vi "Autonomous Independent.vi"   [LabVIEW 2017]
doc: "This VI is called when autonomous begins, and will automatically be terminated when autonomous ends. You can carry out timed or sensor driven robot movement independently without needing to return to the caller."
uses:
  Autonomous/Enum_AutoAction.ctl
  Autonomous/Enum_AutoState.ctl
  Systems/Gear/ENUM_Servo Position.ctl
  Systems/MechamumDrive/Cluster_CMD to SM Data.ctl
  Systems/MechamumDrive/Enum_SM Cmd Select.ctl
  Systems/Shooter/Cluster_CMD to SM Data.ctl
  Systems/Shooter/ENUM_CMD Select.ctl
  Systems/MechamumDrive/Cluster_SM Status.ctl
  Shared Code/TypeDefs/ENUM_Auto Select.ctl
  <vilib>/Rock Robotics/WPI/DriverStation/WPI_DriverStationAllianceInfo.ctl
  Systems/Sonar/Global_HW_Data Out.vi
  Globals/Global_STOP.vi
  Systems/DashBoardCom/Global_Dashboard Controls.vi
  Systems/MechamumDrive/Global_SM Out Data.vi
  Globals/Global_Alliance.vi
  Systems/Shooter/Global_CMD to SM Data.vi
  Systems/MechamumDrive/Global_CMD to SM Data.vi
  Systems/Gear/Global_CMD to HW.vi
  Systems/Hopper/Global_SM_Data Out.vi
  Systems/Gear/Gear.lvlib
  Systems/Sonar/Sonar.lvlib
  Systems/Hopper/Hopper System.lvlib
  Systems/MechamumDrive/MechamunDrive.lvlib
  Systems/DashBoardCom/DashBoardCom.lvlib
  Systems/Shooter/Shooter.lvlib
types:
  T1 = typedef "WPI_DriverStationAllianceInfo.ctl" = enum16{"Red", "Blue", "Invalid"}
  T2 = typedef "ENUM_Auto Select.ctl" = enum16{"None", "Cross Baseline", "Shoot", "Middle Peg", "Right Peg", "Left Peg", "Middle Peg and Shoot", "Side Peg and Shoot", "Dump Hopper and Shoot"}
  T3 = typedef "MechamunDrive.lvlib/Cluster_SM Status.ctl" = cluster{"Drive Cmd":T4, "Complete":bool}
  T4 = typedef "MechamunDrive.lvlib/Enum_SM Cmd Select.ctl" = enum16{"No Command", "Halt", "Manual Keep Rotation", "Manual", "Track Front", "Track Rotation", "Track Lateral", "Track Vision Lat", "Track Vision Rot", "Strafe Right", "Strafe Left"}
  T5 = typedef "Shooter.lvlib/Cluster_CMD to SM Data.ctl" = cluster{"Select":T6, "Wheel VBus":dbl, "Wheel RPM":dbl, "Hood VBus":dbl, "Hood Position":dbl}
  T6 = typedef "Shooter.lvlib/ENUM_CMD Select.ctl" = enum16{"Stop", "Manual VBus", "Encoder Hood Only", "Encoder Wheel Only", "Encoder Both"}
  T7 = typedef "MechamunDrive.lvlib/Cluster_CMD to SM Data.ctl" = cluster{"CMDMODE":T4, "X":dbl, "Y":dbl, "Rotation":dbl, "Auto Angle":dbl, "Speed Divider":dbl, "Use Gyro":bool, "Target Distance":dbl}
  T8 = typedef "Gear.lvlib/ENUM_Servo Position.ctl" = enum16{"Back", "Forward"}
  T9 = typedef "Enum_AutoState.ctl" = enum16{"Startup", "Preparing to Shoot", "Idle", "Shutdown", "Crossing Baseline", "Moving To Boiler", "Rotating To Boiler", "Vision Locking", "Shooting", "Moving to Side Peg", "Placing Gear", "Stalling", "Moving from peg", "Positioning", "Moving to hopper", "Dumping Hopper", "Rotating to Hopper", "Position To Boiler", "Rotating Side Peg"}
  T10 = typedef "Enum_AutoAction.ctl" = enum16{"Stop All", "Reset Time", "Reset All", "No action", "Move Forward", "Move Backward", "Rotate To Boiler", "Stop Movement", "Rotate To target", "Prepare To Shoot", "Fire!", "Cross Line", "Stop Shooting", "rotate from middle peg to boiler", "Dump Hopper", "Rotate To Hopper", "Rotate to side peg"}
  T11 = cluster{"Action":T10[], "State":T9, "Current Time":timestamp, "Start Time":timestamp, "Loop time":u32, "Auto Setting":T2, "Alliance":T1, "CMD_Hopper":dbl, "CMD_Gear":T8, "CMD_Drive":T7, "CMD_Shooter":T5, "Gyro Angle":dbl, "Sonar Distance":dbl, "Drive_SM_Status":T3, "Target Angle":dbl}
  T12 = typedef "Cluster_DashBoard to Rio Controls.ctl" = cluster{"Auto Select":T2}
  T13 = cluster{"Yaw":dbl, "Roll":dbl, "Pitch":dbl, "Heading":dbl, "Fused Heading":dbl}
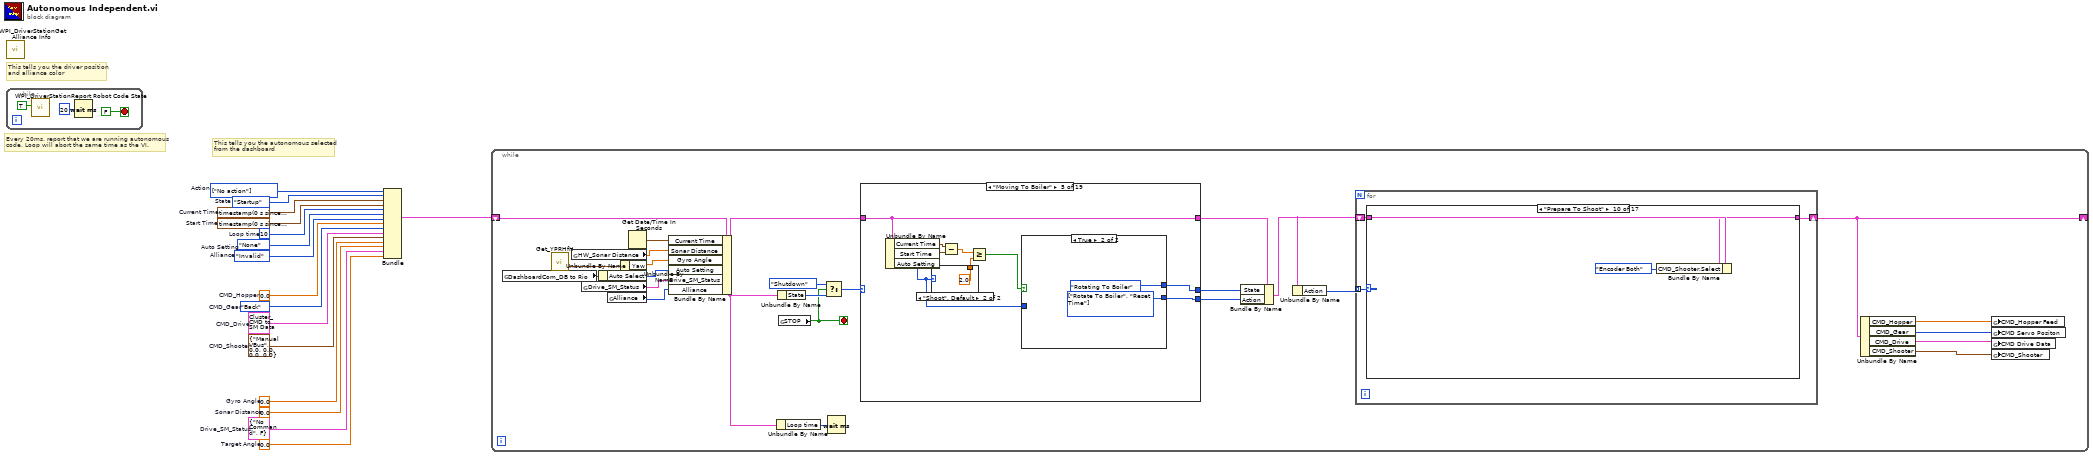
[diagram p0: block diagram]
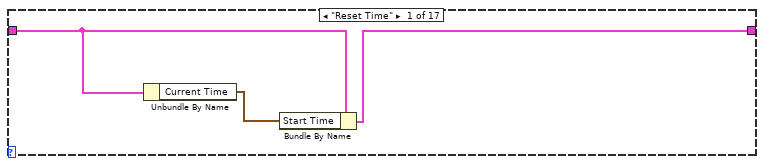
[diagram p2: hidden frame]
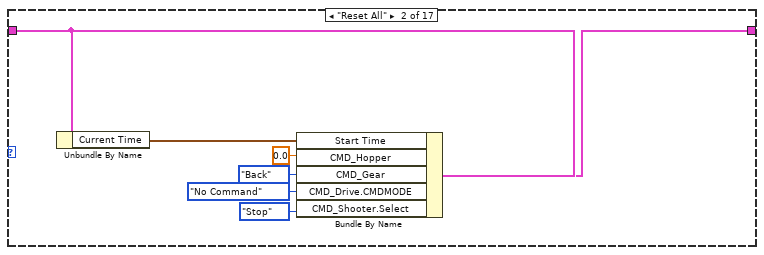
[diagram p3: hidden frame]
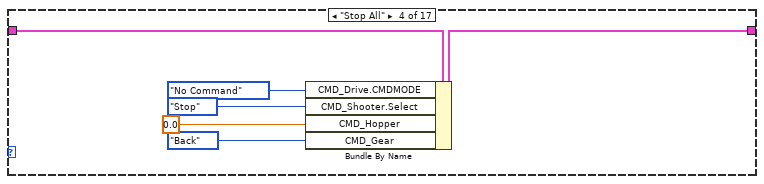
[diagram p5: hidden frame]
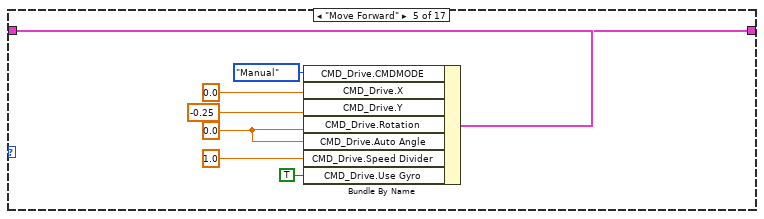
[diagram p6: hidden frame]
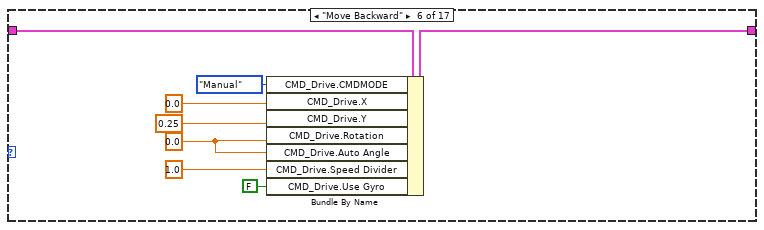
[diagram p7: hidden frame]
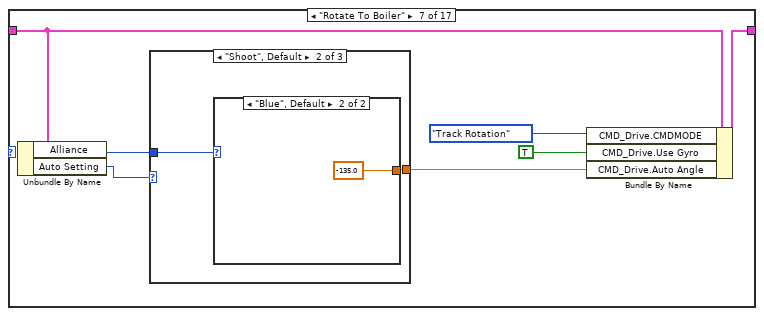
[diagram p8: hidden frame]
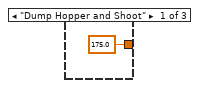
[diagram p9: hidden frame]
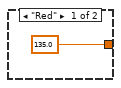
[diagram p10: hidden frame]
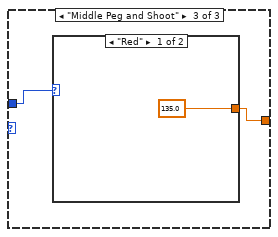
[diagram p11: hidden frame]
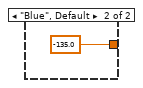
[diagram p12: hidden frame]
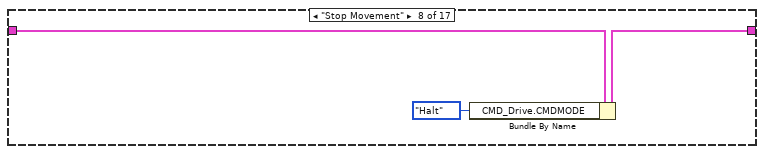
[diagram p13: hidden frame]
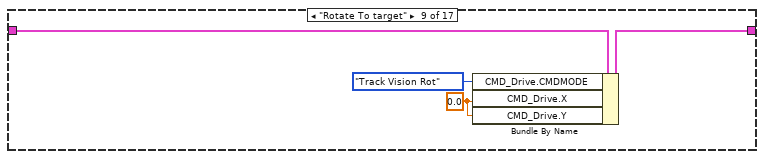
[diagram p14: hidden frame]
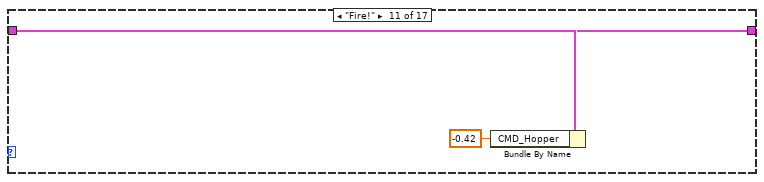
[diagram p15: hidden frame]
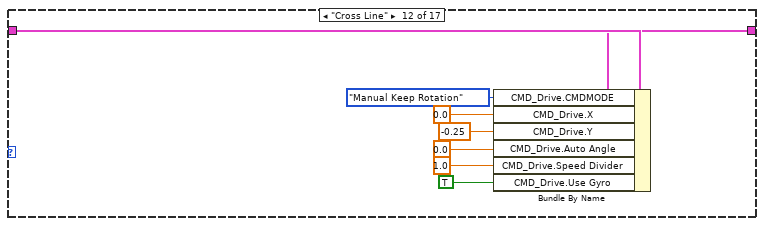
[diagram p16: hidden frame]
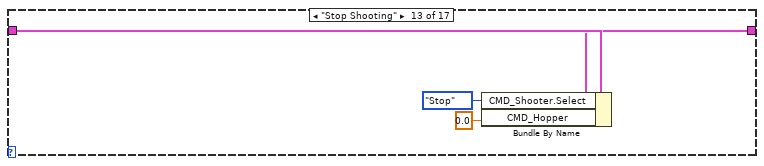
[diagram p17: hidden frame]
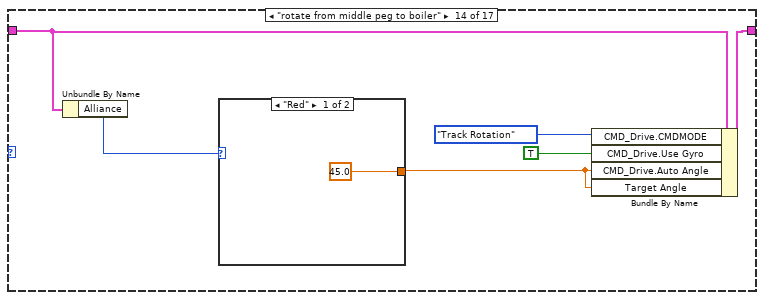
[diagram p18: hidden frame]
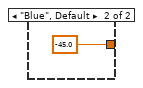
[diagram p19: hidden frame]
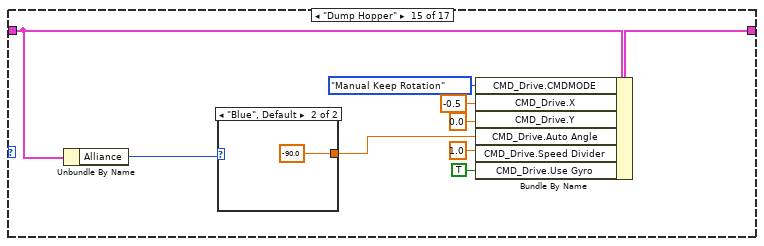
[diagram p20: hidden frame]
diagram:
  w2 = 0.0  # Target Angle
  w10 = WPI_DriverStationAllianceInfo."Invalid"  # Alliance
  w11 = ENUM_Auto_Select."None"  # Auto Setting
  w3 = T3 {"Drive Cmd"=enum."No Command", "Complete"=FALSE}  # Drive_SM_Status
  w6 = T5 {"Select"=enum."Manual VBus", "Wheel VBus"=0.0, "Wheel RPM"=0.0, "Hood VBus"=0.0, "Hood Position"=0.0}  # CMD_Shooter
  w7 = T7 {"CMDMODE"=enum."No Command", "X"=0.0, "Y"=0.0, "Rotation"=0.0, "Auto Angle"=0.0, "Speed Divider"=0.0, "Use Gyro"=FALSE, "Target Distance"=0.0}  # CMD_Drive
  w9 = 0.0  # CMD_Hopper
  w4 = 0.0  # Sonar Distance
  w8 = ENUM_Servo_Position."Back"  # CMD_Gear
  w5 = 0.0  # Gyro Angle
  w12 = u32 10  # Loop time
  w15 = Enum_AutoState."Startup"  # State
  w13 = timestamp(0 s since 1904-01-01)  # Start Time
  w14 = timestamp(0 s since 1904-01-01)  # Current Time
  w16 = T10[] [enum."No action"] items=["Stop All", "Reset Time", "Reset All", "No action", "Move Forward", "Move Backward", "Rotate To Boiler", "Stop Movement", "Rotate To target", "Prepare To Shoot", "Fire!", "Cross Line", "Stop Shooting", "rotate from middle peg to boiler", "Dump Hopper", "Rotate To Hopper", "Rotate to side peg"]  # Action
  # "This tells you the autonomous selected\nfrom the dashboard"
  # "Every 20ms, report that we are running autonomous\ncode. Loop will abort the same time as the VI."
  # "This tells you the driver position\nand alliance color"
  n1 = call <vilib>:"WPI_DriverStationGet Alliance Info.vi"() -> ()  [unwired: 12 out]
  n2 = while {
    stop <- FALSE stop-if-true
    n3 = call <vilib>:"WPI_DriverStationReport Robot Code State.vi"("Autonomous"=TRUE) -> ()  [unwired: 10 in, 1 out]
    n4 = Wait (ms)(milliseconds to wait=u32 20) -> ()  [unwired: 1 out]
  }
  n5 = Bundle("Action"=w16, "State"=w15, "Current Time"=w14, "Start Time"=w13, "Loop time"=w12, "Auto Setting"=w11, "Alliance"=w10, "CMD_Hopper"=w9, "CMD_Gear"=w8, "CMD_Drive"=w7, "CMD_Shooter"=w6, "Gyro Angle"=w5, "Sonar Distance"=w4, "Drive_SM_Status"=w3, "Target Angle"=w2) -> (w1:T11)  [unwired: 1 in]
  n6 = while {
    shift-right: [w39] -> _
    shift-left: w1 -> [w43]
    stop <- w31 stop-if-true
    n7 = global read "Global_Dashboard Controls.vi" "DashboardCom_DB to Rio"() -> (w25:T12)
    n8 = call <vilib>:"Get_YPRHfH.vi"() -> ("YRPHfH"=w44:T13)  [unwired: 11 in]
    n9 = global read "Global_HW_Data Out.vi" "HW_Sonar Distance"() -> (w41:dbl)
    n10 = global read "Global_SM Out Data.vi" "Drive_SM_Status"() -> (w22:T3)
    n11 = Unbundle By Name(w25) -> ("Auto Select"=w21:T2)
    n12 = global read "Global_Alliance.vi" "Alliance"() -> (w20:T1)
    n13 = Unbundle By Name(w44) -> ("Yaw"=w40:dbl)
    n14 = Get Date/Time In Seconds() -> (seconds since 1Jan1904=w42:timestamp)
    n15 = Bundle By Name(cluster=w43, "Current Time"=w42, "Sonar Distance"=w41, "Gyro Angle"=w40, "Auto Setting"=w21, "Drive_SM_Status"=w22, "Alliance"=w20) -> (w33:T11)
    n16 = Unbundle By Name(w33) -> ("Loop time"=w32:u32)
    n17 = Unbundle By Name(w33) -> ("State"=w35:T9)
    n18 = global read "Global_STOP.vi" "STOP"() -> (w31:bool)
    n19 = Select(t=Enum_AutoState."Shutdown", s=w31, f=w35) -> (s? t:f=w36:T9)
    n20 = Wait (ms)(milliseconds to wait=w32) -> ()  [unwired: 1 out]
    n21 = case shown="\"Moving To Boiler\"" w36 {
      tunnel: w33 -> [w167 w171 w192 w200 w213 w220 w243 w258 w272 w289 w302 w317 w329 w339 w347 w357 w369 w374 w386]
      tunnel: [w167 w171 w192 w200 w213 w220 w243 w258 w272 w289 w302 w317 w329 w339 w347 w357 w369 w374 w386] -> w30
      tunnel: [Enum_AutoState."Idle" ("State") w169 Enum_AutoState."Shutdown" ("State") w194 w207 w228 w244 w252 w267 w282 w296 w316 w323 w338 w345 w352 w363 w381 w387] -> w27
      tunnel: [w165 w168 w190 w193 w208 w227 w245 w253 w268 w283 w295 w315 w322 w337 w344 w353 w362 w380 w388] -> w26
      frame "Startup" {
        w165 = T10[] [enum."Reset All"] items=["Stop All", "Reset Time", "Reset All", "No action", "Move Forward", "Move Backward", "Rotate To Boiler", "Stop Movement", "Rotate To target", "Prepare To Shoot", "Fire!", "Cross Line", "Stop Shooting", "rotate from middle peg to boiler", "Dump Hopper", "Rotate To Hopper", "Rotate to side peg"] ("Action")
      }
      frame "Idle" {
        n22 = Unbundle By Name(w171) -> ("Auto Setting"=w170:T2)
        n23 = case shown="\"Shoot\"" w170 {
          tunnel: [Enum_AutoState."Shutdown" ("State") Enum_AutoState."Crossing Baseline" ("State") Enum_AutoState."Moving To Boiler" ("State") Enum_AutoState."Placing Gear" ("State") Enum_AutoState."Placing Gear" ("State") Enum_AutoState."Moving to hopper" ("State") Enum_AutoState."Moving to Side Peg" ("State") Enum_AutoState."Moving to Side Peg" ("State") Enum_AutoState."Moving to Side Peg" ("State")] -> w169
          tunnel: [w172 w174 w176 w178 w181 w182 w184 w186 w188] -> w168
          frame "None", Default {
            w172 = T10[] [enum."Stop All"] items=["Stop All", "Reset Time", "Reset All", "No action", "Move Forward", "Move Backward", "Rotate To Boiler", "Stop Movement", "Rotate To target", "Prepare To Shoot", "Fire!", "Cross Line", "Stop Shooting", "rotate from middle peg to boiler", "Dump Hopper", "Rotate To Hopper", "Rotate to side peg"] ("Action")
          }
          frame "Cross Baseline" {
            w174 = T10[] [enum."Cross Line", enum."Reset Time"] items=["Stop All", "Reset Time", "Reset All", "No action", "Move Forward", "Move Backward", "Rotate To Boiler", "Stop Movement", "Rotate To target", "Prepare To Shoot", "Fire!", "Cross Line", "Stop Shooting", "rotate from middle peg to boiler", "Dump Hopper", "Rotate To Hopper", "Rotate to side peg"] ("Action")
          }
          frame "Shoot" {
            w176 = T10[] [enum."Move Forward", enum."Reset Time"] items=["Stop All", "Reset Time", "Reset All", "No action", "Move Forward", "Move Backward", "Rotate To Boiler", "Stop Movement", "Rotate To target", "Prepare To Shoot", "Fire!", "Cross Line", "Stop Shooting", "rotate from middle peg to boiler", "Dump Hopper", "Rotate To Hopper", "Rotate to side peg"] ("Action")
          }
          frame "Middle Peg" {
            w178 = T10[] [enum."Move Forward"] items=["Stop All", "Reset Time", "Reset All", "No action", "Move Forward", "Move Backward", "Rotate To Boiler", "Stop Movement", "Rotate To target", "Prepare To Shoot", "Fire!", "Cross Line", "Stop Shooting", "rotate from middle peg to boiler", "Dump Hopper", "Rotate To Hopper", "Rotate to side peg"] ("Action")
          }
          frame "Middle Peg and Shoot" {
            w181 = T10[] [enum."Move Forward"] items=["Stop All", "Reset Time", "Reset All", "No action", "Move Forward", "Move Backward", "Rotate To Boiler", "Stop Movement", "Rotate To target", "Prepare To Shoot", "Fire!", "Cross Line", "Stop Shooting", "rotate from middle peg to boiler", "Dump Hopper", "Rotate To Hopper", "Rotate to side peg"] ("Action")
          }
          frame "Dump Hopper and Shoot" {
            w182 = T10[] [enum."Move Forward", enum."Reset Time"] items=["Stop All", "Reset Time", "Reset All", "No action", "Move Forward", "Move Backward", "Rotate To Boiler", "Stop Movement", "Rotate To target", "Prepare To Shoot", "Fire!", "Cross Line", "Stop Shooting", "rotate from middle peg to boiler", "Dump Hopper", "Rotate To Hopper", "Rotate to side peg"] ("Action")
          }
          frame "Right Peg" {
            w184 = T10[] [enum."Move Forward", enum."Reset Time"] items=["Stop All", "Reset Time", "Reset All", "No action", "Move Forward", "Move Backward", "Rotate To Boiler", "Stop Movement", "Rotate To target", "Prepare To Shoot", "Fire!", "Cross Line", "Stop Shooting", "rotate from middle peg to boiler", "Dump Hopper", "Rotate To Hopper", "Rotate to side peg"] ("Action")
          }
          frame "Left Peg" {
            w186 = T10[] [enum."Move Forward", enum."Reset Time"] items=["Stop All", "Reset Time", "Reset All", "No action", "Move Forward", "Move Backward", "Rotate To Boiler", "Stop Movement", "Rotate To target", "Prepare To Shoot", "Fire!", "Cross Line", "Stop Shooting", "rotate from middle peg to boiler", "Dump Hopper", "Rotate To Hopper", "Rotate to side peg"] ("Action")
          }
          frame "Side Peg and Shoot" {
            w188 = T10[] [enum."Move Forward", enum."Reset Time"] items=["Stop All", "Reset Time", "Reset All", "No action", "Move Forward", "Move Backward", "Rotate To Boiler", "Stop Movement", "Rotate To target", "Prepare To Shoot", "Fire!", "Cross Line", "Stop Shooting", "rotate from middle peg to boiler", "Dump Hopper", "Rotate To Hopper", "Rotate to side peg"] ("Action")
          }
        }
      }
      frame "Shutdown" {
        w190 = T10[] [enum."Stop All"] items=["Stop All", "Reset Time", "Reset All", "No action", "Move Forward", "Move Backward", "Rotate To Boiler", "Stop Movement", "Rotate To target", "Prepare To Shoot", "Fire!", "Cross Line", "Stop Shooting", "rotate from middle peg to boiler", "Dump Hopper", "Rotate To Hopper", "Rotate to side peg"] ("Action")
      }
      frame "Crossing Baseline" {
        n24 = Unbundle By Name(w200) -> ("Current Time"=w199:timestamp, "Start Time"=w198:timestamp)
        n25 = Subtract(x=w199, y=w198) -> (x-y=w197:dbl)
        n26 = Greater Or Equal?(x=w197, y=5.0) -> (x >= y?=w195:bool)
        n27 = case shown="False" w195 {
          tunnel: [Enum_AutoState."Crossing Baseline" ("State") Enum_AutoState."Shutdown" ("State")] -> w194
          tunnel: [w201 w203] -> w193
          frame False {
            w201 = T10[] [enum."Cross Line"] items=["Stop All", "Reset Time", "Reset All", "No action", "Move Forward", "Move Backward", "Rotate To Boiler", "Stop Movement", "Rotate To target", "Prepare To Shoot", "Fire!", "Cross Line", "Stop Shooting", "rotate from middle peg to boiler", "Dump Hopper", "Rotate To Hopper", "Rotate to side peg"] ("Action")
          }
          frame True {
            w203 = T10[] [enum."Stop All"] items=["Stop All", "Reset Time", "Reset All", "No action", "Move Forward", "Move Backward", "Rotate To Boiler", "Stop Movement", "Rotate To target", "Prepare To Shoot", "Fire!", "Cross Line", "Stop Shooting", "rotate from middle peg to boiler", "Dump Hopper", "Rotate To Hopper", "Rotate to side peg"] ("Action")
          }
        }
      }
      frame "Moving To Boiler" {
        n28 = Unbundle By Name(w213) -> ("Current Time"=w212:timestamp, "Start Time"=w211:timestamp, "Auto Setting"=w205:T2)
        n29 = case shown="\"Shoot\", Default" w205 {
          tunnel: [4.0 ("y") 2.0 ("y")] -> w209
          frame "Middle Peg and Shoot" {
          }
          frame "Shoot", Default {
          }
        }
        n30 = Subtract(x=w212, y=w211) -> (x-y=w210:dbl)
        n31 = Greater Or Equal?(x=w210, y=w209) -> (x >= y?=w206:bool)
        n32 = case shown="True" w206 {
          tunnel: [w217 w218] -> w208
          tunnel: [Enum_AutoState."Moving To Boiler" ("State") Enum_AutoState."Rotating To Boiler" ("State")] -> w207
          tunnel: w205 -> [_ _]
          frame False {
            w217 = T10[] [enum."Move Forward"] items=["Stop All", "Reset Time", "Reset All", "No action", "Move Forward", "Move Backward", "Rotate To Boiler", "Stop Movement", "Rotate To target", "Prepare To Shoot", "Fire!", "Cross Line", "Stop Shooting", "rotate from middle peg to boiler", "Dump Hopper", "Rotate To Hopper", "Rotate to side peg"] ("Action")
          }
          frame True {
            w218 = T10[] [enum."Rotate To Boiler", enum."Reset Time"] items=["Stop All", "Reset Time", "Reset All", "No action", "Move Forward", "Move Backward", "Rotate To Boiler", "Stop Movement", "Rotate To target", "Prepare To Shoot", "Fire!", "Cross Line", "Stop Shooting", "rotate from middle peg to boiler", "Dump Hopper", "Rotate To Hopper", "Rotate to side peg"] ("Action")
          }
        }
      }
      frame "Rotating To Boiler" {
        n33 = Unbundle By Name(w220) -> ("Current Time"=w225:timestamp, "Start Time"=w224:timestamp)
        n34 = Unbundle By Name(w220) -> ("Auto Setting"=w226:T2)
        n35 = Subtract(x=w225, y=w224) -> (x-y=w223:dbl)
        n36 = Greater Or Equal?(x=w223, y=1.5) -> (x >= y?=w221:bool)
        n37 = case shown="True" w221 {
          tunnel: [Enum_AutoState."Rotating To Boiler" ("State") w233] -> w228
          tunnel: [w230 w232] -> w227
          tunnel: w226 -> [_ w231]
          frame False {
            w230 = T10[] [enum."Rotate To Boiler"] items=["Stop All", "Reset Time", "Reset All", "No action", "Move Forward", "Move Backward", "Rotate To Boiler", "Stop Movement", "Rotate To target", "Prepare To Shoot", "Fire!", "Cross Line", "Stop Shooting", "rotate from middle peg to boiler", "Dump Hopper", "Rotate To Hopper", "Rotate to side peg"] ("Action")
          }
          frame True {
            n38 = case shown="\"Shoot\", Default" w231 {
              tunnel: [Enum_AutoState."Position To Boiler" ("State") Enum_AutoState."Preparing to Shoot" ("State")] -> w233
              tunnel: [w234 w236] -> w232
              frame "Middle Peg and Shoot" {
                w234 = T10[] [enum."Move Forward", enum."Reset Time", enum."Prepare To Shoot"] items=["Stop All", "Reset Time", "Reset All", "No action", "Move Forward", "Move Backward", "Rotate To Boiler", "Stop Movement", "Rotate To target", "Prepare To Shoot", "Fire!", "Cross Line", "Stop Shooting", "rotate from middle peg to boiler", "Dump Hopper", "Rotate To Hopper", "Rotate to side peg"] ("Action")
              }
              frame "Shoot", Default {
                w236 = T10[] [enum."Stop Movement", enum."Prepare To Shoot", enum."Reset Time"] items=["Stop All", "Reset Time", "Reset All", "No action", "Move Forward", "Move Backward", "Rotate To Boiler", "Stop Movement", "Rotate To target", "Prepare To Shoot", "Fire!", "Cross Line", "Stop Shooting", "rotate from middle peg to boiler", "Dump Hopper", "Rotate To Hopper", "Rotate to side peg"] ("Action")
              }
            }
          }
        }
      }
      frame "Vision Locking" {
        n39 = Unbundle By Name(w243) -> ("Current Time"=w241:timestamp, "Start Time"=w242:timestamp)
        n40 = Subtract(x=w241, y=w242) -> (x-y=w240:dbl)
        n41 = Greater Or Equal?(x=w240, y=0.5) -> (x >= y?=w238:bool)
        n42 = case shown="True" w238 {
          tunnel: [w246 w249] -> w245
          tunnel: [Enum_AutoState."Vision Locking" ("State") Enum_AutoState."Shooting" ("State")] -> w244
          frame False {
            w246 = T10[] [enum."Rotate To target", enum."Prepare To Shoot"] items=["Stop All", "Reset Time", "Reset All", "No action", "Move Forward", "Move Backward", "Rotate To Boiler", "Stop Movement", "Rotate To target", "Prepare To Shoot", "Fire!", "Cross Line", "Stop Shooting", "rotate from middle peg to boiler", "Dump Hopper", "Rotate To Hopper", "Rotate to side peg"] ("Action")
          }
          frame True {
            w249 = T10[] [enum."Stop Movement", enum."Reset Time", enum."Prepare To Shoot", enum."Fire!"] items=["Stop All", "Reset Time", "Reset All", "No action", "Move Forward", "Move Backward", "Rotate To Boiler", "Stop Movement", "Rotate To target", "Prepare To Shoot", "Fire!", "Cross Line", "Stop Shooting", "rotate from middle peg to boiler", "Dump Hopper", "Rotate To Hopper", "Rotate to side peg"] ("Action")
          }
        }
      }
      frame "Shooting" {
        n43 = Unbundle By Name(w258) -> ("Current Time"=w257:timestamp, "Start Time"=w256:timestamp, "Auto Setting"=w250:T2)
        n44 = case shown="\"Shoot\", Default" w250 {
          tunnel: [10.0 ("y") 6.0 ("y") 6.0 ("y")] -> w254
          frame "Dump Hopper and Shoot" {
          }
          frame "Shoot", Default {
          }
          frame "Middle Peg and Shoot" {
          }
        }
        n45 = Subtract(x=w257, y=w256) -> (x-y=w255:dbl)
        n46 = Greater Or Equal?(x=w255, y=w254) -> (x >= y?=w251:bool)
        n47 = case shown="False" w251 {
          tunnel: [w262 w265] -> w253
          tunnel: [Enum_AutoState."Shooting" ("State") Enum_AutoState."Crossing Baseline" ("State")] -> w252
          frame False {
            w262 = T10[] [enum."Prepare To Shoot", enum."Stop Movement", enum."Fire!"] items=["Stop All", "Reset Time", "Reset All", "No action", "Move Forward", "Move Backward", "Rotate To Boiler", "Stop Movement", "Rotate To target", "Prepare To Shoot", "Fire!", "Cross Line", "Stop Shooting", "rotate from middle peg to boiler", "Dump Hopper", "Rotate To Hopper", "Rotate to side peg"] ("Action")
          }
          frame True {
            w265 = T10[] [enum."Cross Line", enum."Stop Shooting"] items=["Stop All", "Reset Time", "Reset All", "No action", "Move Forward", "Move Backward", "Rotate To Boiler", "Stop Movement", "Rotate To target", "Prepare To Shoot", "Fire!", "Cross Line", "Stop Shooting", "rotate from middle peg to boiler", "Dump Hopper", "Rotate To Hopper", "Rotate to side peg"] ("Action")
          }
        }
      }
      frame "Placing Gear" {
        n48 = Unbundle By Name(w272) -> ("Sonar Distance"=w271:dbl, "Auto Setting"=w266:T2)
        n49 = Less Or Equal?(x=w271, y=22.0) -> (x <= y?=w269:bool)
        n50 = case shown="True" w269 {
          tunnel: [w273 w277] -> w268
          tunnel: [Enum_AutoState."Placing Gear" ("State") w276] -> w267
          tunnel: w266 -> [_ w275]
          frame False {
            w273 = T10[] [enum."Move Forward"] items=["Stop All", "Reset Time", "Reset All", "No action", "Move Forward", "Move Backward", "Rotate To Boiler", "Stop Movement", "Rotate To target", "Prepare To Shoot", "Fire!", "Cross Line", "Stop Shooting", "rotate from middle peg to boiler", "Dump Hopper", "Rotate To Hopper", "Rotate to side peg"] ("Action")
          }
          frame True {
            n51 = case shown="\"Left Peg\", Default" w275 {
              tunnel: [w278 w281] -> w277
              tunnel: [Enum_AutoState."Shutdown" ("State") Enum_AutoState."Shutdown" ("State")] -> w276
              frame "Middle Peg" {
                w278 = T10[] [enum."Stop Movement", enum."Reset Time"] items=["Stop All", "Reset Time", "Reset All", "No action", "Move Forward", "Move Backward", "Rotate To Boiler", "Stop Movement", "Rotate To target", "Prepare To Shoot", "Fire!", "Cross Line", "Stop Shooting", "rotate from middle peg to boiler", "Dump Hopper", "Rotate To Hopper", "Rotate to side peg"] ("Action")
              }
              frame "Left Peg", Default {
                w281 = T10[] [enum."Stop Movement", enum."Reset Time"] items=["Stop All", "Reset Time", "Reset All", "No action", "Move Forward", "Move Backward", "Rotate To Boiler", "Stop Movement", "Rotate To target", "Prepare To Shoot", "Fire!", "Cross Line", "Stop Shooting", "rotate from middle peg to boiler", "Dump Hopper", "Rotate To Hopper", "Rotate to side peg"] ("Action")
              }
            }
          }
        }
      }
      frame "Stalling" {
        n52 = Unbundle By Name(w289) -> ("Current Time"=w288:timestamp, "Start Time"=w287:timestamp)
        n53 = Subtract(x=w288, y=w287) -> (x-y=w286:dbl)
        n54 = Greater Or Equal?(x=w286, y=2.0) -> (x >= y?=w284:bool)
        n55 = case shown="True" w284 {
          tunnel: [w291 w293] -> w283
          tunnel: [Enum_AutoState."Stalling" ("State") Enum_AutoState."Moving from peg" ("State")] -> w282
          frame False {
            w291 = T10[] [enum."Stop Movement"] items=["Stop All", "Reset Time", "Reset All", "No action", "Move Forward", "Move Backward", "Rotate To Boiler", "Stop Movement", "Rotate To target", "Prepare To Shoot", "Fire!", "Cross Line", "Stop Shooting", "rotate from middle peg to boiler", "Dump Hopper", "Rotate To Hopper", "Rotate to side peg"] ("Action")
          }
          frame True {
            w293 = T10[] [enum."Move Backward", enum."Reset Time"] items=["Stop All", "Reset Time", "Reset All", "No action", "Move Forward", "Move Backward", "Rotate To Boiler", "Stop Movement", "Rotate To target", "Prepare To Shoot", "Fire!", "Cross Line", "Stop Shooting", "rotate from middle peg to boiler", "Dump Hopper", "Rotate To Hopper", "Rotate to side peg"] ("Action")
          }
        }
      }
      frame "Moving from peg" {
        n56 = Unbundle By Name(w302) -> ("Current Time"=w301:timestamp, "Start Time"=w300:timestamp, "Auto Setting"=w294:T2)
        n57 = Subtract(x=w301, y=w300) -> (x-y=w299:dbl)
        n58 = Greater Or Equal?(x=w299, y=2.0) -> (x >= y?=w297:bool)
        n59 = case shown="True" w297 {
          tunnel: [Enum_AutoState."Moving from peg" ("State") w306] -> w296
          tunnel: [w303 w305] -> w295
          tunnel: w294 -> [_ w307]
          frame False {
            w303 = T10[] [enum."Move Backward"] items=["Stop All", "Reset Time", "Reset All", "No action", "Move Forward", "Move Backward", "Rotate To Boiler", "Stop Movement", "Rotate To target", "Prepare To Shoot", "Fire!", "Cross Line", "Stop Shooting", "rotate from middle peg to boiler", "Dump Hopper", "Rotate To Hopper", "Rotate to side peg"] ("Action")
          }
          frame True {
            n60 = case shown="\"Side Peg and Shoot\"" w307 {
              tunnel: [Enum_AutoState."Shutdown" ("State") Enum_AutoState."Positioning" ("State") Enum_AutoState."Rotating To Boiler" ("State")] -> w306
              tunnel: [w308 w311 w312] -> w305
              frame "None", Default {
                w308 = T10[] [enum."Stop All"] items=["Stop All", "Reset Time", "Reset All", "No action", "Move Forward", "Move Backward", "Rotate To Boiler", "Stop Movement", "Rotate To target", "Prepare To Shoot", "Fire!", "Cross Line", "Stop Shooting", "rotate from middle peg to boiler", "Dump Hopper", "Rotate To Hopper", "Rotate to side peg"] ("Action")
              }
              frame "Middle Peg and Shoot" {
                w311 = T10[] [enum."rotate from middle peg to boiler"] items=["Stop All", "Reset Time", "Reset All", "No action", "Move Forward", "Move Backward", "Rotate To Boiler", "Stop Movement", "Rotate To target", "Prepare To Shoot", "Fire!", "Cross Line", "Stop Shooting", "rotate from middle peg to boiler", "Dump Hopper", "Rotate To Hopper", "Rotate to side peg"] ("Action")
              }
              frame "Side Peg and Shoot" {
                w312 = T10[] [enum."Rotate To Boiler", enum."Reset Time"] items=["Stop All", "Reset Time", "Reset All", "No action", "Move Forward", "Move Backward", "Rotate To Boiler", "Stop Movement", "Rotate To target", "Prepare To Shoot", "Fire!", "Cross Line", "Stop Shooting", "rotate from middle peg to boiler", "Dump Hopper", "Rotate To Hopper", "Rotate to side peg"] ("Action")
              }
            }
          }
        }
      }
      frame "Positioning" {
        n61 = Unbundle By Name(w317) -> ("Drive_SM_Status.Complete"=w314:bool)
        n62 = case shown="True" w314 {
          tunnel: [Enum_AutoState."Positioning" ("State") Enum_AutoState."Moving To Boiler" ("State")] -> w316
          tunnel: [w318 w321] -> w315
          frame False {
            w318 = T10[] [enum."rotate from middle peg to boiler"] items=["Stop All", "Reset Time", "Reset All", "No action", "Move Forward", "Move Backward", "Rotate To Boiler", "Stop Movement", "Rotate To target", "Prepare To Shoot", "Fire!", "Cross Line", "Stop Shooting", "rotate from middle peg to boiler", "Dump Hopper", "Rotate To Hopper", "Rotate to side peg"] ("Action")
          }
          frame True {
            w321 = T10[] [enum."Move Forward", enum."Reset Time"] items=["Stop All", "Reset Time", "Reset All", "No action", "Move Forward", "Move Backward", "Rotate To Boiler", "Stop Movement", "Rotate To target", "Prepare To Shoot", "Fire!", "Cross Line", "Stop Shooting", "rotate from middle peg to boiler", "Dump Hopper", "Rotate To Hopper", "Rotate to side peg"] ("Action")
          }
        }
      }
      frame "Moving to hopper" {
        n63 = Unbundle By Name(w329) -> ("Current Time"=w328:timestamp, "Start Time"=w327:timestamp)
        n64 = Subtract(x=w328, y=w327) -> (x-y=w326:dbl)
        n65 = Greater Or Equal?(x=w326, y=3.0) -> (x >= y?=w324:bool)
        n66 = case shown="True" w324 {
          tunnel: [Enum_AutoState."Moving to hopper" ("State") Enum_AutoState."Rotating to Hopper" ("State")] -> w323
          tunnel: [w330 w332] -> w322
          frame False {
            w330 = T10[] [enum."Move Forward"] items=["Stop All", "Reset Time", "Reset All", "No action", "Move Forward", "Move Backward", "Rotate To Boiler", "Stop Movement", "Rotate To target", "Prepare To Shoot", "Fire!", "Cross Line", "Stop Shooting", "rotate from middle peg to boiler", "Dump Hopper", "Rotate To Hopper", "Rotate to side peg"] ("Action")
          }
          frame True {
            w332 = T10[] [enum."Rotate To Hopper", enum."Reset Time"] items=["Stop All", "Reset Time", "Reset All", "No action", "Move Forward", "Move Backward", "Rotate To Boiler", "Stop Movement", "Rotate To target", "Prepare To Shoot", "Fire!", "Cross Line", "Stop Shooting", "rotate from middle peg to boiler", "Dump Hopper", "Rotate To Hopper", "Rotate to side peg"] ("Action")
          }
        }
      }
      frame "Dumping Hopper" {
        n67 = Unbundle By Name(w339) -> ("Sonar Distance"=w336:dbl)
        n68 = Less Or Equal?(x=w336, y=30.0) -> (x <= y?=w334:bool)
        n69 = case shown="True" w334 {
          tunnel: [Enum_AutoState."Dumping Hopper" ("State") Enum_AutoState."Rotating To Boiler" ("State")] -> w338
          tunnel: [w340 w342] -> w337
          frame False {
            w340 = T10[] [enum."Move Forward"] items=["Stop All", "Reset Time", "Reset All", "No action", "Move Forward", "Move Backward", "Rotate To Boiler", "Stop Movement", "Rotate To target", "Prepare To Shoot", "Fire!", "Cross Line", "Stop Shooting", "rotate from middle peg to boiler", "Dump Hopper", "Rotate To Hopper", "Rotate to side peg"] ("Action")
          }
          frame True {
            w342 = T10[] [enum."Rotate To Boiler"] items=["Stop All", "Reset Time", "Reset All", "No action", "Move Forward", "Move Backward", "Rotate To Boiler", "Stop Movement", "Rotate To target", "Prepare To Shoot", "Fire!", "Cross Line", "Stop Shooting", "rotate from middle peg to boiler", "Dump Hopper", "Rotate To Hopper", "Rotate to side peg"] ("Action")
          }
        }
      }
      frame "Rotating to Hopper" {
        n70 = Unbundle By Name(w347) -> ("Drive_SM_Status.Complete"=w346:bool)
        n71 = case shown="True" w346 {
          tunnel: [Enum_AutoState."Rotating to Hopper" ("State") Enum_AutoState."Dumping Hopper" ("State")] -> w345
          tunnel: [w349 w350] -> w344
          frame False {
            w349 = T10[] [enum."Rotate To Hopper"] items=["Stop All", "Reset Time", "Reset All", "No action", "Move Forward", "Move Backward", "Rotate To Boiler", "Stop Movement", "Rotate To target", "Prepare To Shoot", "Fire!", "Cross Line", "Stop Shooting", "rotate from middle peg to boiler", "Dump Hopper", "Rotate To Hopper", "Rotate to side peg"] ("Action")
          }
          frame True {
            w350 = T10[] [enum."Move Forward"] items=["Stop All", "Reset Time", "Reset All", "No action", "Move Forward", "Move Backward", "Rotate To Boiler", "Stop Movement", "Rotate To target", "Prepare To Shoot", "Fire!", "Cross Line", "Stop Shooting", "rotate from middle peg to boiler", "Dump Hopper", "Rotate To Hopper", "Rotate to side peg"] ("Action")
          }
        }
      }
      frame "Position To Boiler" {
        n72 = Unbundle By Name(w357) -> ("Sonar Distance"=w355:dbl)
        n73 = Less Or Equal?(x=w355, y=90.0) -> (x <= y?=w354:bool)
        n74 = case shown="True" w354 {
          tunnel: [w359 w361] -> w353
          tunnel: [Enum_AutoState."Position To Boiler" ("State") Enum_AutoState."Vision Locking" ("State")] -> w352
          frame False {
            w359 = T10[] [enum."Move Forward"] items=["Stop All", "Reset Time", "Reset All", "No action", "Move Forward", "Move Backward", "Rotate To Boiler", "Stop Movement", "Rotate To target", "Prepare To Shoot", "Fire!", "Cross Line", "Stop Shooting", "rotate from middle peg to boiler", "Dump Hopper", "Rotate To Hopper", "Rotate to side peg"] ("Action")
          }
          frame True {
            w361 = T10[] [enum."Rotate To target", enum."Reset Time"] items=["Stop All", "Reset Time", "Reset All", "No action", "Move Forward", "Move Backward", "Rotate To Boiler", "Stop Movement", "Rotate To target", "Prepare To Shoot", "Fire!", "Cross Line", "Stop Shooting", "rotate from middle peg to boiler", "Dump Hopper", "Rotate To Hopper", "Rotate to side peg"] ("Action")
          }
        }
      }
      frame "Moving to Side Peg" {
        n75 = Unbundle By Name(w369) -> ("Current Time"=w368:timestamp, "Start Time"=w367:timestamp)
        n76 = Subtract(x=w368, y=w367) -> (x-y=w366:dbl)
        n77 = Greater Or Equal?(x=w366, y=3.25) -> (x >= y?=w364:bool)
        n78 = case shown="True" w364 {
          tunnel: [Enum_AutoState."Moving to Side Peg" ("State") Enum_AutoState."Rotating Side Peg" ("State")] -> w363
          tunnel: [w370 w372] -> w362
          frame False {
            w370 = T10[] [enum."Move Forward"] items=["Stop All", "Reset Time", "Reset All", "No action", "Move Forward", "Move Backward", "Rotate To Boiler", "Stop Movement", "Rotate To target", "Prepare To Shoot", "Fire!", "Cross Line", "Stop Shooting", "rotate from middle peg to boiler", "Dump Hopper", "Rotate To Hopper", "Rotate to side peg"] ("Action")
          }
          frame True {
            w372 = T10[] [enum."Rotate to side peg", enum."Reset Time"] items=["Stop All", "Reset Time", "Reset All", "No action", "Move Forward", "Move Backward", "Rotate To Boiler", "Stop Movement", "Rotate To target", "Prepare To Shoot", "Fire!", "Cross Line", "Stop Shooting", "rotate from middle peg to boiler", "Dump Hopper", "Rotate To Hopper", "Rotate to side peg"] ("Action")
          }
        }
      }
      frame "Rotating Side Peg" {
        n79 = Unbundle By Name(w374) -> ("Current Time"=w379:timestamp, "Start Time"=w378:timestamp)
        n80 = Subtract(x=w379, y=w378) -> (x-y=w377:dbl)
        n81 = Greater Or Equal?(x=w377, y=1.5) -> (x >= y?=w375:bool)
        n82 = case shown="True" w375 {
          tunnel: [Enum_AutoState."Rotating Side Peg" ("State") Enum_AutoState."Placing Gear" ("State")] -> w381
          tunnel: [w382 w384] -> w380
          frame False {
            w382 = T10[] [enum."Rotate to side peg"] items=["Stop All", "Reset Time", "Reset All", "No action", "Move Forward", "Move Backward", "Rotate To Boiler", "Stop Movement", "Rotate To target", "Prepare To Shoot", "Fire!", "Cross Line", "Stop Shooting", "rotate from middle peg to boiler", "Dump Hopper", "Rotate To Hopper", "Rotate to side peg"] ("Action")
          }
          frame True {
            w384 = T10[] [enum."Move Forward"] items=["Stop All", "Reset Time", "Reset All", "No action", "Move Forward", "Move Backward", "Rotate To Boiler", "Stop Movement", "Rotate To target", "Prepare To Shoot", "Fire!", "Cross Line", "Stop Shooting", "rotate from middle peg to boiler", "Dump Hopper", "Rotate To Hopper", "Rotate to side peg"] ("Action")
          }
        }
      }
      frame "Preparing to Shoot" {
        n83 = Unbundle By Name(w386) -> ("Current Time"=w393:timestamp, "Start Time"=w392:timestamp)
        n84 = Subtract(x=w393, y=w392) -> (x-y=w391:dbl)
        n85 = Greater Or Equal?(x=w391, y=2.0) -> (x >= y?=w389:bool)
        n86 = case shown="True" w389 {
          tunnel: [w395 w396] -> w388
          tunnel: [Enum_AutoState."Preparing to Shoot" ("State") Enum_AutoState."Shooting" ("State")] -> w387
          frame False {
            w395 = T10[] [enum."Prepare To Shoot"] items=["Stop All", "Reset Time", "Reset All", "No action", "Move Forward", "Move Backward", "Rotate To Boiler", "Stop Movement", "Rotate To target", "Prepare To Shoot", "Fire!", "Cross Line", "Stop Shooting", "rotate from middle peg to boiler", "Dump Hopper", "Rotate To Hopper", "Rotate to side peg"] ("Action")
          }
          frame True {
            w396 = T10[] [enum."Prepare To Shoot", enum."Fire!", enum."Reset Time"] items=["Stop All", "Reset Time", "Reset All", "No action", "Move Forward", "Move Backward", "Rotate To Boiler", "Stop Movement", "Rotate To target", "Prepare To Shoot", "Fire!", "Cross Line", "Stop Shooting", "rotate from middle peg to boiler", "Dump Hopper", "Rotate To Hopper", "Rotate to side peg"] ("Action")
          }
        }
      }
    }
    n87 = Bundle By Name(cluster=w30, "State"=w27, "Action"=w26) -> (w29:T11)
    n88 = Unbundle By Name(w29) -> ("Action"=w28:T10[])
    n89 = for {
      shift-right: [w46] -> w39
      shift-left: w29 -> [w47]
      tunnel: w28 -> [w45] mode=indexing
      n90 = case shown="\"Prepare To Shoot\"" w45 {
        tunnel: w47 -> [w50 w57 w58 w64 w72 w74 w86 w99 w103 w106 w109 w117 w121 w124 w137 w142 w154]
        tunnel: [w49 w56 w58 w63 w71 w73 w85 w98 w102 w105 w108 w116 w120 w123 w136 w141 w153] -> w46
        frame "Reset Time" {
          n91 = Unbundle By Name(w50) -> ("Current Time"=w48:timestamp)
          n92 = Bundle By Name(cluster=w50, "Start Time"=w48) -> (w49:T11)
        }
        frame "Reset All" {
          n93 = Unbundle By Name(w57) -> ("Current Time"=w55:timestamp)
          n94 = Bundle By Name(cluster=w57, "Start Time"=w55, "CMD_Hopper"=0.0, "CMD_Gear"=ENUM_Servo_Position."Back", "CMD_Drive.CMDMODE"=Enum_SM_Cmd_Select."No Command", "CMD_Shooter.Select"=ENUM_CMD_Select."Stop") -> (w56:T11)
        }
        frame "No action" {
        }
        frame "Stop All" {
          n95 = Bundle By Name(cluster=w64, "CMD_Drive.CMDMODE"=Enum_SM_Cmd_Select."No Command" ("Drive Data.CMDMODE"), "CMD_Shooter.Select"=ENUM_CMD_Select."Stop", "CMD_Hopper"=0.0 ("Hopper Feed"), "CMD_Gear"=ENUM_Servo_Position."Back") -> (w63:T11)
        }
        frame "Move Forward" {
          w67 = 0.0 ("CMD_Drive.Rotation")
          n96 = Bundle By Name(cluster=w72, "CMD_Drive.CMDMODE"=Enum_SM_Cmd_Select."Manual", "CMD_Drive.X"=0.0, "CMD_Drive.Y"=-0.25, "CMD_Drive.Rotation"=w67, "CMD_Drive.Auto Angle"=w67, "CMD_Drive.Speed Divider"=1.0, "CMD_Drive.Use Gyro"=TRUE) -> (w71:T11)
        }
        frame "Move Backward" {
          w77 = 0.0 ("CMD_Drive.Rotation")
          n97 = Bundle By Name(cluster=w74, "CMD_Drive.CMDMODE"=Enum_SM_Cmd_Select."Manual", "CMD_Drive.X"=0.0, "CMD_Drive.Y"=0.25, "CMD_Drive.Rotation"=w77, "CMD_Drive.Auto Angle"=w77, "CMD_Drive.Speed Divider"=1.0, "CMD_Drive.Use Gyro"=FALSE) -> (w73:T11)
        }
        frame "Rotate To Boiler" {
          n98 = Unbundle By Name(w86) -> ("Alliance"=w87:T1, "Auto Setting"=w81:T2)
          n99 = case shown="\"Shoot\", Default" w81 {
            tunnel: w87 -> [_ w90 w94]
            tunnel: [175.0 ("CMD_Drive.Auto Angle") w89 w93] -> w82
            frame "Dump Hopper and Shoot" {
            }
            frame "Shoot", Default {
              n100 = case shown="\"Blue\", Default" w90 {
                tunnel: [135.0 ("CMD_Drive.Auto Angle") -135.0 ("CMD_Drive.Auto Angle")] -> w89
                frame "Red" {
                }
                frame "Blue", Default {
                }
              }
            }
            frame "Middle Peg and Shoot" {
              n101 = case shown="\"Red\"" w94 {
                tunnel: [135.0 ("CMD_Drive.Auto Angle") -135.0 ("CMD_Drive.Auto Angle")] -> w93
                frame "Red" {
                }
                frame "Blue", Default {
                }
              }
            }
          }
          n102 = Bundle By Name(cluster=w86, "CMD_Drive.CMDMODE"=Enum_SM_Cmd_Select."Track Rotation", "CMD_Drive.Use Gyro"=TRUE, "CMD_Drive.Auto Angle"=w82) -> (w85:T11)
        }
        frame "Stop Movement" {
          n103 = Bundle By Name(cluster=w99, "CMD_Drive.CMDMODE"=Enum_SM_Cmd_Select."Halt") -> (w98:T11)
        }
        frame "Rotate To target" {
          w100 = 0.0 ("CMD_Drive.X")
          n104 = Bundle By Name(cluster=w103, "CMD_Drive.CMDMODE"=Enum_SM_Cmd_Select."Track Vision Rot", "CMD_Drive.X"=w100, "CMD_Drive.Y"=w100) -> (w102:T11)
        }
        frame "Prepare To Shoot" {
          n105 = Bundle By Name(cluster=w106, "CMD_Shooter.Select"=ENUM_CMD_Select."Encoder Both") -> (w105:T11)
        }
        frame "Fire!" {
          n106 = Bundle By Name(cluster=w109, "CMD_Hopper"=-0.42) -> (w108:T11)
        }
        frame "Cross Line" {
          n107 = Bundle By Name(cluster=w117, "CMD_Drive.CMDMODE"=Enum_SM_Cmd_Select."Manual Keep Rotation", "CMD_Drive.X"=0.0, "CMD_Drive.Y"=-0.25, "CMD_Drive.Auto Angle"=0.0, "CMD_Drive.Speed Divider"=1.0 ("CMD_Drive.Auto Angle"), "CMD_Drive.Use Gyro"=TRUE) -> (w116:T11)
        }
        frame "Stop Shooting" {
          n108 = Bundle By Name(cluster=w121, "CMD_Shooter.Select"=ENUM_CMD_Select."Stop", "CMD_Hopper"=0.0) -> (w120:T11)
        }
        frame "rotate from middle peg to boiler" {
          n109 = Unbundle By Name(w124) -> ("Alliance"=w127:T1)
          n110 = case shown="\"Red\"" w127 {
            tunnel: [45.0 ("CMD_Drive.Auto Angle") -45.0 ("CMD_Drive.Auto Angle")] -> w122
            frame "Red" {
            }
            frame "Blue", Default {
            }
          }
          n111 = Bundle By Name(cluster=w124, "CMD_Drive.CMDMODE"=Enum_SM_Cmd_Select."Track Rotation", "CMD_Drive.Use Gyro"=TRUE, "CMD_Drive.Auto Angle"=w122, "Target Angle"=w122) -> (w123:T11)
        }
        frame "Dump Hopper" {
          n112 = Unbundle By Name(w137) -> ("Alliance"=w138:T1)
          n113 = case shown="\"Blue\", Default" w138 {
            tunnel: [90.0 ("CMD_Drive.Auto Angle") -90.0 ("CMD_Drive.Auto Angle")] -> w132
            frame "Red" {
            }
            frame "Blue", Default {
            }
          }
          n114 = Bundle By Name(cluster=w137, "CMD_Drive.CMDMODE"=Enum_SM_Cmd_Select."Manual Keep Rotation", "CMD_Drive.X"=-0.5, "CMD_Drive.Y"=0.0, "CMD_Drive.Auto Angle"=w132, "CMD_Drive.Speed Divider"=1.0, "CMD_Drive.Use Gyro"=TRUE) -> (w136:T11)
        }
        frame "Rotate To Hopper" {
          n115 = Unbundle By Name(w142) -> ("Alliance"=w149:T1)
          n116 = case shown="\"Blue\", Default" w149 {
            tunnel: [90.0 ("CMD_Drive.Auto Angle") -90.0 ("CMD_Drive.Auto Angle")] -> w145
            frame "Red" {
            }
            frame "Blue", Default {
            }
          }
          n117 = Bundle By Name(cluster=w142, "CMD_Drive.CMDMODE"=Enum_SM_Cmd_Select."Track Rotation", "CMD_Drive.X"=0.0, "CMD_Drive.Y"=0.0, "CMD_Drive.Auto Angle"=w145, "CMD_Drive.Speed Divider"=1.0, "CMD_Drive.Use Gyro"=TRUE) -> (w141:T11)
        }
        frame "Rotate to side peg" {
          n118 = Unbundle By Name(w154) -> ("Auto Setting"=w158:T2, "Alliance"=w157:T1)
          n119 = case shown="\"Right Peg\"" w158 {
            tunnel: w157 -> [_ w161 _]
            tunnel: [60.0 ("CMD_Drive.Y") w160 -60.0 ("CMD_Drive.Y")] -> w152
            frame "Left Peg" {
            }
            frame "Side Peg and Shoot", Default {
              n120 = case shown="\"Red\"" w161 {
                tunnel: [-60.0 ("CMD_Drive.Y") 60.0 ("CMD_Drive.Y")] -> w160
                frame "Red" {
                }
                frame "Blue", Default {
                }
              }
            }
            frame "Right Peg" {
            }
          }
          n121 = Bundle By Name(cluster=w154, "CMD_Drive.CMDMODE"=Enum_SM_Cmd_Select."Track Rotation", "CMD_Drive.Use Gyro"=TRUE, "CMD_Drive.Auto Angle"=w152) -> (w153:T11)
        }
      }
    }
    n122 = Unbundle By Name(w39) -> ("CMD_Hopper"=w37:dbl, "CMD_Gear"=w38:T8, "CMD_Drive"=w24:T7, "CMD_Shooter"=w23:T5)
    n123 = global write "Global_SM_Data Out.vi" "CMD_Hopper Feed"(w37) -> ()
    n124 = global write "Global_CMD to HW.vi" "CMD Servo Positon"(w38) -> ()
    n125 = global write "Global_CMD to SM Data.vi" "CMD Drive Data"(w24) -> ()
    n126 = global write "Global_CMD to SM Data.vi" "CMD_Shooter"(w23) -> ()
  }
